vi "Create Subset Buffers.vi"(6 "inline buffer offset":u64 format="%d bytes", 7 "string buffer offset":u64 format="%d bytes", 8 "error in (no error)":errorcluster, 9 "inline buffer size":u64 format="%d bytes", 10 "string buffer size":u64 format="%d bytes", 11 "Transfer Group in":refnum<class "Transfer Group.lvclass">) -> (0 "error out":errorcluster, 2 "subset Buffers":refnum<class "Buffers.lvclass">, 3 "Transfer Group out":refnum<class "Transfer Group.lvclass">, 4 "inline buffer offset +size":u64 format="%d bytes", 5 "string buffer offset + size":u64 format="%d bytes")   [LabVIEW 2021, in "DSF Core.lvlib" / "Transfer Group.lvclass"]
uses:
  Transfer Group.lvclass
  Buffers/Buffers.lvclass
  Transfer Group.lvclass/Transfer Group.ctl
  Buffers/Buffers.lvclass/Buffers.ctl
  <vilib>/NI/Memory Manager/Classes/Pointer/Pointer.lvclass/Pointer.ctl
  Buffer/Buffer.lvclass/Buffer.ctl
  Buffer/Subset Buffer.vi
  <vilib>/Utility/error.llb/Clear Errors.vi
  Buffer/Set Buffer Size.vi
  Buffers/Create.vi
  <vilib>/NI/Memory Manager/Classes/Pointer/Subset.vi
  Buffer/Set Buffer Offset.vi
  <vilib>/NI/Memory Manager/Classes/Pointer/Set Size.vi
  <vilib>/NI/Memory Manager/Classes/Pointer/Get Address.vi
  <vilib>/NI/Memory Manager/Classes/Pointer/Encapsulate.vi
  <vilib>/NI/Memory Manager/Classes/Pointer/Check Null Pointer.vi
  <vilib>/NI/Memory Manager/Classes/Pointer/Check Length.vi
  <vilib>/NI/Memory Manager/Classes/Pointer/Set Address.vi
  <vilib>/NI/Memory Manager/Classes/Pointer/Set Internal.vi
  <vilib>/NI/Memory Manager/Classes/Pointer/Errors.vi
  <vilib>/NI/Memory Manager/Classes/Pointer/Null Pointer.vi
  <vilib>/NI/Memory Manager/Classes/Pointer/Is Null.vi
  <vilib>/NI/Memory Manager/Classes/Pointer/Get Size.vi
  <vilib>/NI/Memory Manager/Classes/Pointer/Check Bounds (Pointer).vi
  <vilib>/NI/Memory Manager/Classes/Pointer/Create Error.vi
  <vilib>/NI/Memory Manager/Classes/Pointer/Out of Bounds.vi
  <vilib>/NI/Memory Manager/VIs/New Error Cluster.vi
  <vilib>/NI/Memory Manager/VIs/New Error Cluster (512B).vi
  <vilib>/NI/Memory Manager/VIs/Set Error Status.vi
  <vilib>/NI/Memory Manager/VIs/Set Error Code.vi
  <vilib>/NI/Memory Manager/VIs/Set Error Source.vi
  <vilib>/NI/Memory Manager/Constants/Constants.vi
  <vilib>/NI/Memory Manager/Constants/Library Name.vi
  <vilib>/NI/Memory Manager/Classes/Pointer/Pointer Error Info.vi
  <vilib>/NI/Memory Manager/VIs/Write String to Source.vi
  <vilib>/NI/Memory Manager/Constants/Pointer Class Name.vi
  <vilib>/NI/Memory Manager/Classes/Pointer/Write Pointer Size to Error.vi
  <vilib>/NI/Memory Manager/VIs/Write Numeric to Source.vi
  <vilib>/NI/Memory Manager/VIs/Write Numeric Scalar to Source (Base10 U64).vi
  Buffer/Buffer.lvclass
  C:/Program Files/National Instruments/LabVIEW 2021/vi.lib/NI/Memory Manager/Classes/Pointer/Pointer.lvclass
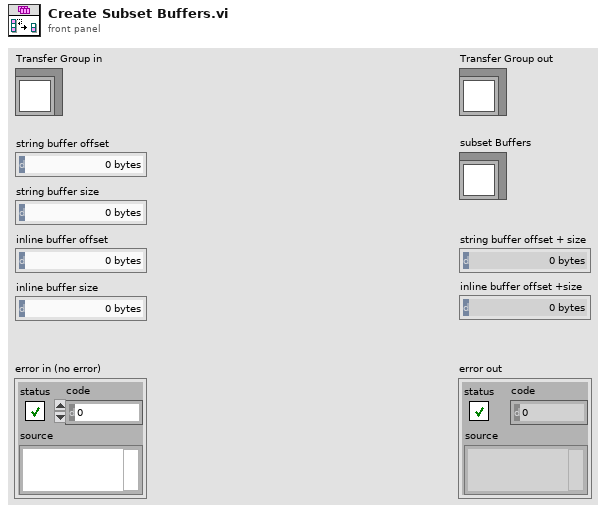
[diagram p1: front panel]
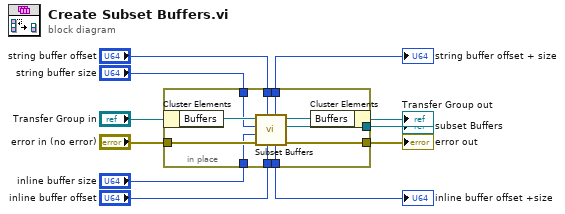
[diagram p0: block diagram]
diagram:
  n1 = in-place {
    in-place-border: "error in (no error)" -> [w22]
    in-place-border: [w21] -> w10
    in-place-border: [w20] -> w9
    in-place-border: "inline buffer size" -> [w17]
    in-place-border: "string buffer size" -> [w16]
    in-place-border: "string buffer offset" -> [w15]
    in-place-border: "inline buffer offset" -> [w14]
    in-place-border: [w13] -> w2
    in-place-border: [w12] -> w1
    n2 = in-place-cluster #1("Transfer Group in") -> ("Buffers"=w19:refnum<class "Buffers.lvclass">)
    n3 = call "Subset Buffers.vi"("engine buffer offset"=w14, "string buffer offset"=w15, "error in (no error)"=w22, "engine buffer size"=w17, "string buffer size"=w16, "Buffers in"=w19) -> ("error out"=w20:errorcluster, "subset Buffers"=w21:refnum<class "Buffers.lvclass">, "Buffers out"=w18:refnum<class "Buffers.lvclass">, "engine buffer offset +size"=w12:u64, "string buffer offset + size"=w13:u64)  [unwired: 1 in]
    n4 = in-place-cluster #1("Buffers"=w18) -> (→"Transfer Group out":refnum<class "Transfer Group.lvclass">)
  }
  "error out" <- w9
  "subset Buffers" <- w10
  "string buffer offset + size" <- w2
  "inline buffer offset +size" <- w1
